vi "ForceBalanceServer.vi"() -> ()   [LabVIEW 2017]
uses:
  <vilib>/Analysis/4window.llb/windowTd.ctl
  <vilib>/measure/maspectr.llb/Power Spectrum and PSD Export Mode.ctl
  <vilib>/Analysis/baseanly.llb/Mean (DBL).vi
  <vilib>/Analysis/baseanly.llb/A x Vector.vi
  Globals/mainWTControl.vi
  <vilib>/Utility/file.llb/Write To Spreadsheet File (DBL).vi
  <vilib>/Utility/file.llb/Read From Spreadsheet File (DBL).vi
  <vilib>/measure/maspectr.llb/FFT Power Spectrum and PSD for 1 Chan.vi
  <vilib>/Analysis/NI_AALBase.lvlib
  <vilib>/measure/NI_MAPro.lvlib
  <vilib>/Analysis/NI_AALPro.lvlib
panel:
  out "PSD":cluster{"f0":dbl, "df":dbl, "magnitude":dbl[]}(graph)
  in  "Time Target (s)":dbl=100000.0
  in  "Sampling Period":dbl=0.01
  in  "Sampling Freq.":dbl=500.0
  in  "x":bool
  out "Fx                     Fy                     Fz                    Mx                   My                    Mz":dbl[](array[numeric])=[0.39367133033328505, 0.12640519158271346, -0.035168369141984894, 0.07356448847559971, 0.08928756090020755, 0.03408632169703757]
  in  "stop":bool
  out "Waveform Chart":dynamicdata(graph)=[{"t0"=timestamp(3625740071.8186145 s since 1904-01-01), "dt"=0.002, "Y"=[1.4132434446437658, 1.4869062871436736, 1.4652020568354351, 1.4342899711432204, 1.515516408827019], "attributes"=variant("NI_ChannelName"=variant(string "Voltage_0"), "NI_UnitDescription"=variant(string "Volts"))}, {"t0"=timestamp(3625740071.8186283 s since 1904-01-01), "dt"=0.002, "Y"=[0.4493782119596065, 0.441156910799936, 0.42537201251587176, 0.4112313744050537, 0.41221793055431444], "attributes"=variant("NI_ChannelName"=variant(string "Voltage_1"), "NI_UnitDescription"=variant(string "Volts"))}, {"t0"=timestamp(3625740071.818642 s since 1904-01-01), "dt"=0.002, "Y"=[0.1241435215364698, 0.13861301307479987, 0.18070607894651378, 0.13466678811720997, 0.12841859858966923], "attributes"=variant("NI_ChannelName"=variant(string "Voltage_2"), "NI_UnitDescription"=variant(string "Volts"))}, {"t0"=timestamp(3625740071.8186564 s since 1904-01-01), "dt"=0.002, "Y"=[4.929329220143692, 4.876055168157049, 4.92110791573665, 4.952020020475538, 4.8872361419192885], "attributes"=variant("NI_ChannelName"=variant(string "Voltage_3"), "NI_UnitDescription"=variant(string "Volts"))}, {"t0"=timestamp(3625740071.8186703 s since 1904-01-01), "dt"=0.002, "Y"=[1.7019754755920375, 1.6973715480570852, 1.6858617292118738, 1.741437711535304, 1.7019754755920375], "attributes"=variant("NI_ChannelName"=variant(string "Voltage_4"), "NI_UnitDescription"=variant(string "Volts"))}, {"t0"=timestamp(3625740071.8186846 s since 1904-01-01), "dt"=0.002, "Y"=[-1.6523161496933905, -1.626994516567589, -1.6023305886073516, -1.6164712405886696, -1.6292964831977657], "attributes"=variant("NI_ChannelName"=variant(string "Voltage_5"), "NI_UnitDescription"=variant(string "Volts"))}]
  out "L2                   S                  D2                  L1                  L3                  D1":dbl[](array[numeric])=[1.4630316337186229, 0.42787128804695646, 0.14130960005293253, 1.7057243879976673, 4.913149693286444, -1.6254817957309533]
  out "Amber Check":bool[](array[boolean])
  out "Amber Check Fail":bool
  out "OMFG Check":bool[](array[boolean])
  out "OMFG Check Fail":bool
  out "Mean Convergence":dbl(graph)=0.08995560655426219
  in  "Blank Button":bool
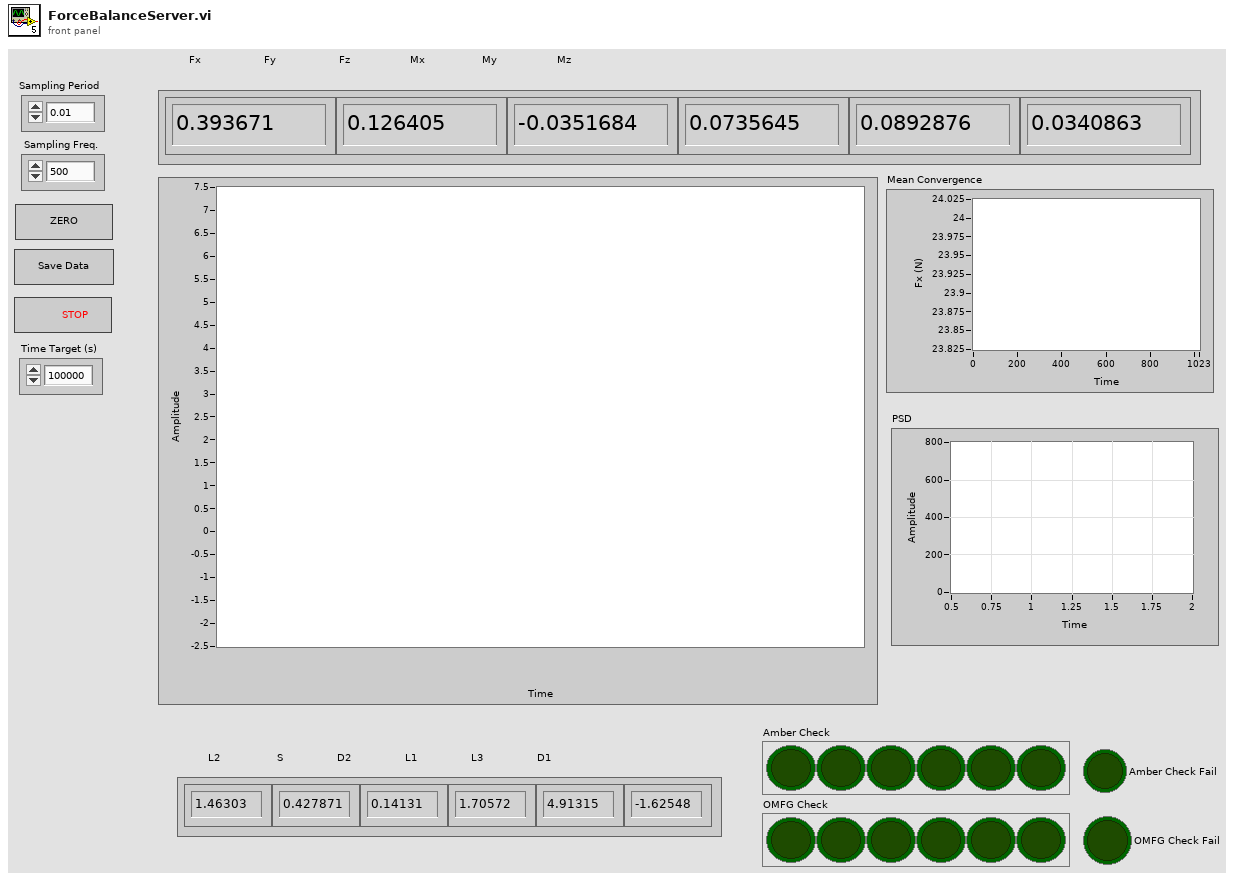
[diagram p1: front panel]
types:
  T1 = typedef "NI_MAPro.lvlib/Power Spectrum and PSD Export Mode.ctl" = u16
  T2 = typedef "NI_AALPro.lvlib/windowTd.ctl" = u32
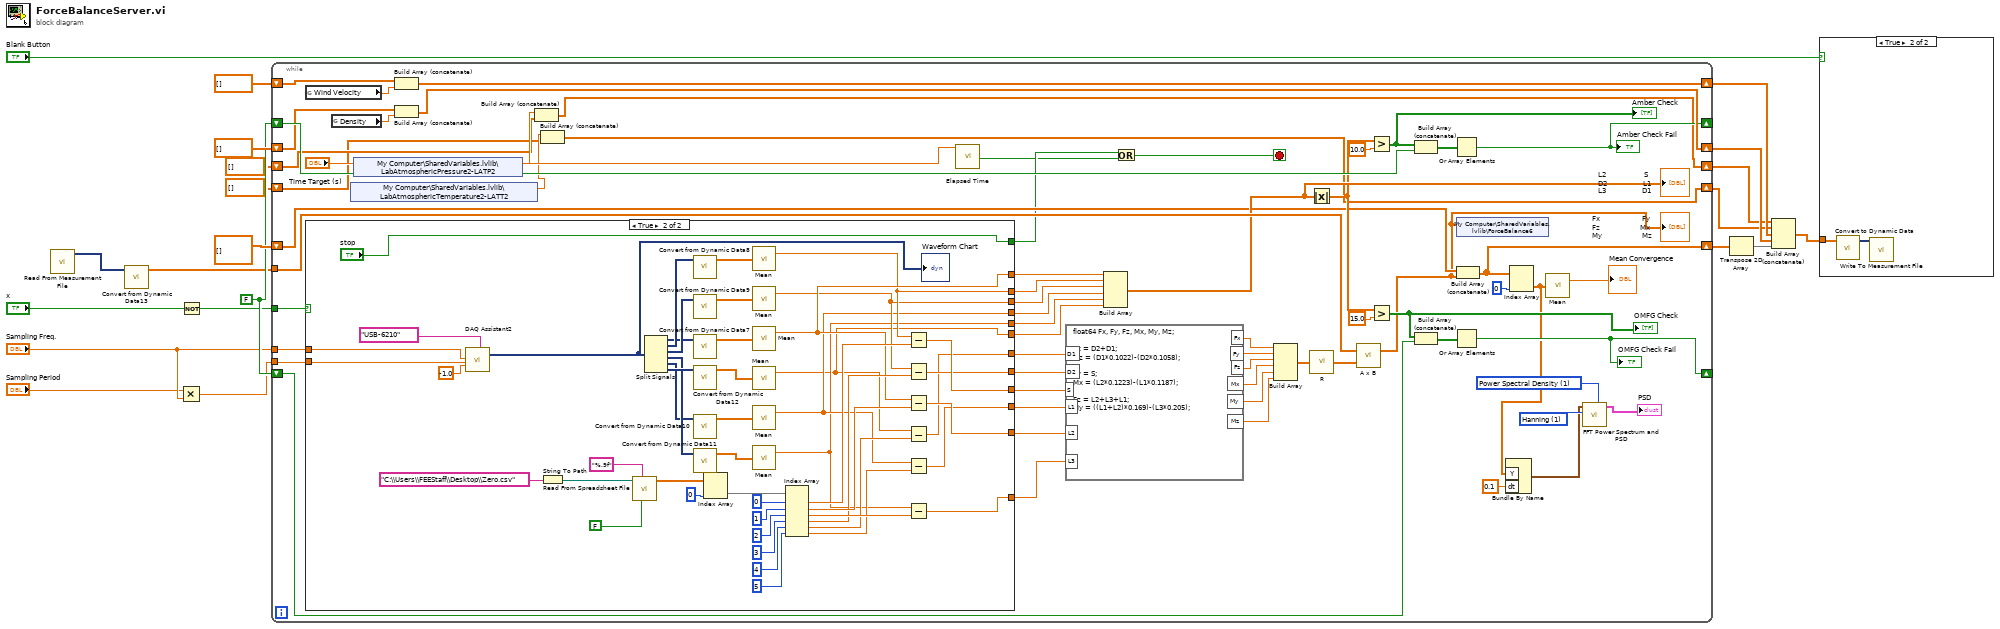
[diagram p0: block diagram]
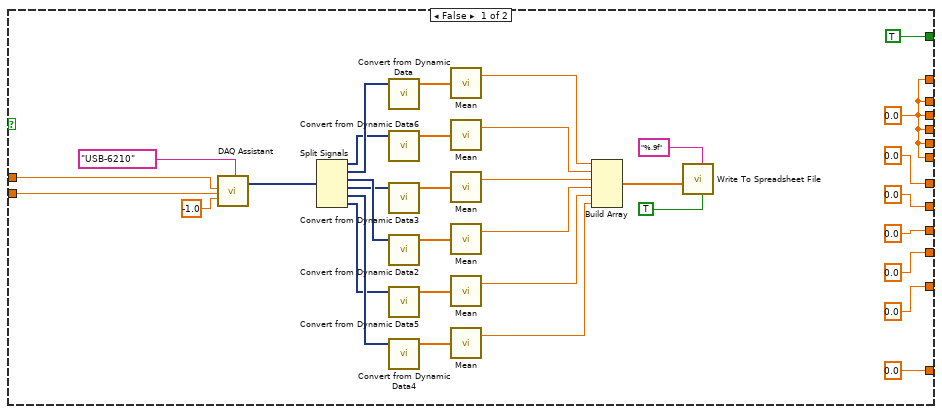
[diagram p3: hidden frame]
diagram:
  w13 = FALSE
  n1 = call "Read From Measurement File"() -> ("Signals"=w10:dynamicdata)  [unwired: 6 in, 5 out]
  n2 = call "Convert from Dynamic Data13"("Dynamic Data Type"=w10) -> ("Array"=w11:dbl[][])  [unwired: 3 in]
  n3 = Multiply(x="Sampling Period", y="Sampling Freq.") -> (x*y=w9:dbl)
  n4 = Not(x="x") -> (.not. x?=w5:bool)
  n5 = while {
    tunnel: w5 -> [w84]
    tunnel: "Sampling Freq." -> [w83]
    tunnel: w9 -> [w82]
    tunnel: w11 -> [w81]
    shift-right: [w40] -> _
    shift-left: w13 -> [w58]
    shift-right: [w41] -> _
    shift-left: w13 -> [w53]
    shift-right: [w49] -> w18
    shift-left: dbl[] [] -> [w48]
    shift-right: [w46] -> w16
    shift-left: dbl[] [] -> [w45]
    shift-right: [w42] -> w19
    shift-left: dbl[][] [] -> [w43]
    shift-right: [w31] -> w2
    shift-left: dbl[] [] -> [w32]
    shift-right: [w30] -> w1
    shift-left: dbl[] [] -> [w29]
    stop <- w36 stop-if-true
    w26 = T1 1 items=["Power Spectrum", "Power Spectral Density"] ("export mode")
    w27 = T2 1 items=["Rectangle"=0, "Hanning"=1, "Hamming"=2, "Blackman-Harris"=3, "Exact Blackman"=4, "Blackman"=5, "Flat Top"=6, "4 Term B-Harris "=7, "7 Term B-Harris"=8, "Low Sidelobe"=9, "Blackman Nuttall"=11, "Triangle"=30, "Bartlett-Hanning"=31, "Bohman"=32, "Parzen"=33, "Welch"=34, "Kaiser"=60, "Dolph-Chebyshev"=61, "Gaussian"=62] ("window")
    n6 = global read "mainWTControl.vi" "Wind Velocity"() -> (w50:dbl)
    n7 = case shown="True" w84 {
      tunnel: [0.0 w133] -> w74
      tunnel: [0.0 w132] -> w73
      tunnel: [0.0 w152] -> w77
      tunnel: [0.0 w151] -> w76
      tunnel: [0.0 w153] -> w75
      tunnel: [0.0 w154] -> w78
      tunnel: w83 -> [w118 w167]
      tunnel: w82 -> [w117 w166]
      tunnel: [TRUE ("stop") "stop"] -> w38
      tunnel: [w85 w124] -> w66
      tunnel: [w85 w123] -> w65
      tunnel: [w85 w122] -> w64
      tunnel: [w85 w121] -> w63
      tunnel: [w85 w120] -> w62
      tunnel: [w85 w119] -> w61
      frame False {
        w85 = 0.0
        n8 = call "DAQ Assistant"("rate"=w118, "number of samples"=w117, "timeout (s)"=-1.0, "device name"=tag "USB-6210") -> ("data"=w104:dynamicdata)  [unwired: 13 in, 2 out]
        n9 = Split Signals(w104) -> (w92:dynamicdata, w103:dynamicdata, w101:dynamicdata, w99:dynamicdata, w97:dynamicdata, w95:dynamicdata)  [unwired: 6 in]
        n10 = call "Convert from Dynamic Data"("Dynamic Data Type"=w103) -> ("Array"=w102:dbl[])  [unwired: 3 in]
        n11 = call "Convert from Dynamic Data6"("Dynamic Data Type"=w92) -> ("Array"=w88:dbl[])  [unwired: 3 in]
        n12 = call "Convert from Dynamic Data3"("Dynamic Data Type"=w99) -> ("Array"=w98:dbl[])  [unwired: 3 in]
        n13 = call "Convert from Dynamic Data2"("Dynamic Data Type"=w101) -> ("Array"=w100:dbl[])  [unwired: 3 in]
        n14 = call "Convert from Dynamic Data5"("Dynamic Data Type"=w95) -> ("Array"=w94:dbl[])  [unwired: 3 in]
        n15 = call "Convert from Dynamic Data4"("Dynamic Data Type"=w97) -> ("Array"=w96:dbl[])  [unwired: 3 in]
        n16 = call-poly <vilib>:"Mean.vi"("X"=w102) -> ("mean"=w109:dbl)  [unwired: 1 out]
        n17 = call-poly <vilib>:"Mean.vi"("X"=w88) -> ("mean"=w106:dbl)  [unwired: 1 out]
        n18 = call-poly <vilib>:"Mean.vi"("X"=w98) -> ("mean"=w89:dbl)  [unwired: 1 out]
        n19 = call-poly <vilib>:"Mean.vi"("X"=w100) -> ("mean"=w108:dbl)  [unwired: 1 out]
        n20 = call-poly <vilib>:"Mean.vi"("X"=w94) -> ("mean"=w107:dbl)  [unwired: 1 out]
        n21 = call-poly <vilib>:"Mean.vi"("X"=w96) -> ("mean"=w87:dbl)  [unwired: 1 out]
        n22 = Build Array(w109, w106, w89, w108, w107, w87) -> (w105:dbl[])
        n23 = call-poly <vilib>:"Write To Spreadsheet File.vi"("transpose? (no:F)"=TRUE, "format (%.3f)"="%.9f", "1D data"=w105) -> ()  [unwired: 5 in, 1 out]
      }
      frame True {
        n24 = call "DAQ Assistant2"("rate"=w167, "number of samples"=w166, "timeout (s)"=-1.0, "device name"=tag "USB-6210") -> ("data"=w125:dynamicdata)  [unwired: 12 in, 3 out]
        "Waveform Chart" <- w125
        n25 = String To Path(string="C:\\Users\\FEEStaff\\Desktop\\Zero.csv" ("format (%.3f)")) -> (path=w134:path)
        n26 = call-poly <vilib>:"Read From Spreadsheet File.vi"("transpose (no:F)"=FALSE, "format (%.3f)"="%.9f", "file path (dialog if empty)"=w134) -> ("all rows"=w157:dbl[][])  [unwired: 4 in, 4 out]
        n27 = Split Signals(w125) -> (w141:dynamicdata, w147:dynamicdata, w145:dynamicdata, w128:dynamicdata, w127:dynamicdata, w142:dynamicdata)  [unwired: 6 in]
        n28 = call "Convert from Dynamic Data8"("Dynamic Data Type"=w147) -> ("Array"=w146:dbl[])  [unwired: 3 in]
        n29 = call "Convert from Dynamic Data9"("Dynamic Data Type"=w145) -> ("Array"=w130:dbl[])  [unwired: 3 in]
        n30 = call "Convert from Dynamic Data7"("Dynamic Data Type"=w141) -> ("Array"=w148:dbl[])  [unwired: 3 in]
        n31 = call "Convert from Dynamic Data12"("Dynamic Data Type"=w142) -> ("Array"=w131:dbl[])  [unwired: 3 in]
        n32 = call "Convert from Dynamic Data10"("Dynamic Data Type"=w127) -> ("Array"=w144:dbl[])  [unwired: 3 in]
        n33 = call "Convert from Dynamic Data11"("Dynamic Data Type"=w128) -> ("Array"=w143:dbl[])  [unwired: 3 in]
        n34 = Index Array(array=w157, index (col)=0 ("disabled index (col)")) -> (element=w155:dbl[])  [unwired: 1 in]
        n35 = call-poly <vilib>:"Mean.vi"("X"=w146) -> ("mean"=w123:dbl)  [unwired: 1 out]
        n36 = call-poly <vilib>:"Mean.vi"("X"=w130) -> ("mean"=w122:dbl)  [unwired: 1 out]
        n37 = call-poly <vilib>:"Mean.vi"("X"=w148) -> ("mean"=w124:dbl)  [unwired: 1 out]
        n38 = call-poly <vilib>:"Mean.vi"("X"=w131) -> ("mean"=w119:dbl)  [unwired: 1 out]
        n39 = call-poly <vilib>:"Mean.vi"("X"=w144) -> ("mean"=w121:dbl)  [unwired: 1 out]
        n40 = call-poly <vilib>:"Mean.vi"("X"=w143) -> ("mean"=w120:dbl)  [unwired: 1 out]
        n41 = Index Array(array=w155, index #1=0 ("index (row)"), index #2=1 ("index (row)"), index #3=2 ("index (row)"), index #4=3 ("index (row)"), index #5=4 ("index (row)"), index #6=5 ("index (row)")) -> (element #1=w140:dbl, element #2=w139:dbl, element #3=w138:dbl, element #4=w137:dbl, element #5=w136:dbl, element #6=w129:dbl)
        n42 = Subtract(x=w123, y=w140) -> (x-y=w154:dbl)
        n43 = Subtract(x=w122, y=w137) -> (x-y=w133:dbl)
        n44 = Subtract(x=w124, y=w139) -> (x-y=w152:dbl)
        n45 = Subtract(x=w119, y=w136) -> (x-y=w132:dbl)
        n46 = Subtract(x=w121, y=w129) -> (x-y=w151:dbl)
        n47 = Subtract(x=w120, y=w138) -> (x-y=w153:dbl)
      }
    }
    n48 = global read "mainWTControl.vi" "Density"() -> (w47:dbl)
    n49 = shared-variable "My Computer\\SharedVariables.lvlib\\LabAtmosphericTemperature2-LATT2"() -> (w33:dbl)  [unwired: 1 in, 1 out]
    n50 = shared-variable "My Computer\\SharedVariables.lvlib\\LabAtmosphericPressure2-LATP2"() -> (w34:dbl)  [unwired: 1 in, 1 out]
    n51 = Build Array (concatenate)(w48, w50) -> (w49:dbl[])
    n52 = Build Array (concatenate)(w45, w47) -> (w46:dbl[])
    n53 = Build Array (concatenate)(w34, w32) -> (w31:dbl[])
    n54 = Build Array (concatenate)(w33, w29) -> (w30:dbl[])
    n55 = call "Elapsed Time"("Time Target (s)"="Time Target (s)") -> ("Time has Elapsed"=w37:bool)  [unwired: 11 in, 7 out]
    n56 = formula code="float64 Fx, Fy, Fz, Mx, My, Mz;\n\nFx = D2+D1;\nMz = (D1*0.1022)-(D2*0.1058);\n\nFy = S;\nMx = (L2*0.1223)-(L1*0.1187);\n\nFz = L2+L3+L1;\nMy = ((L1+L2)*0.169)-(L3*0.205);"("D1"=w73, "D2"=w74, "S"=w78, "L1"=w76, "L2"=w77, "L3"=w75) -> ("Fx"=w72:dbl, "Fy"=w71:dbl, "Fz"=w70:dbl, "Mx"=w69:dbl, "My"=w68:dbl, "Mz"=w67:dbl)
    n57 = Build Array(w66, w65, w64, w63, w62, w61) -> (w60:dbl[])
    "L2                   S                  D2                  L1                  L3                  D1" <- w60
    n58 = Or(x=w38, y=w37) -> (x .or. y?=w36:bool)
    n59 = Build Array(w72, w71, w70, w69, w68, w67) -> (w79:dbl[])
    n60 = Absolute Value(x=w60) -> (abs(x)=w55:dbl[])
    n61 = call "R.vi"("1x6"=w79) -> ("27x1"=w80:dbl[])
    n62 = call-poly <vilib>:"A x B.vi"("Vector"=w80, "A"=w81) -> ("A x Vector"=w39:dbl[])  [unwired: 1 out]
    "Fx                     Fy                     Fz                    Mx                   My                    Mz" <- w39
    n63 = Greater?(x=w55, y=10.0 ("Numeric")) -> (0:w56:bool[])
    "Amber Check" <- w56
    n64 = Greater?(x=w55, y=15.0) -> (0:w51:bool[])
    "OMFG Check" <- w51
    n65 = Build Array (concatenate)(w56, w58) -> (w57:bool[])
    n66 = Build Array (concatenate)(w51, w53) -> (w52:bool[])
    n67 = Or Array Elements(Boolean array=w57) -> (logical OR=w40:bool)
    "Amber Check Fail" <- w40
    n68 = Or Array Elements(Boolean array=w52) -> (logical OR=w41:bool)
    "OMFG Check Fail" <- w41
    n69 = shared-variable "My Computer\\SharedVariables.lvlib\\ForceBalance6"(w39) -> ()  [unwired: 1 in, 1 out]
    n70 = Build Array (concatenate)(w43, w39) -> (w42:dbl[][])
    n71 = Index Array(array=w42, index (col)=0 ("index")) -> (element=w24:dbl[])  [unwired: 1 in]
    n72 = Bundle By Name("Y"=w24, "dt"=0.1) -> (w22:waveform(dbl))  [unwired: 1 in]
    n73 = call-poly <vilib>:"Mean.vi"("X"=w24) -> ("mean"=→"Mean Convergence":dbl)  [unwired: 1 out]
    n74 = call-poly <vilib>:"FFT Power Spectrum and PSD.vi"("export mode"=w26, "window"=w27, "time signal"=w22) -> ("Power Spectrum / PSD"=→"PSD":cluster{"f0":dbl, "df":dbl, "magnitude":dbl[]})  [unwired: 5 in, 3 out]
  }
  n75 = Transpose 2D Array(2D array=w19) -> (transposed array=w20:dbl[][])
  n76 = Build Array (concatenate)(w2, w1, w18, w16, w20) -> (w21:dbl[][])
  n77 = case shown="True" "Blank Button" {
    tunnel: w21 -> [_ w169]
    frame False {
    }
    frame True {
      n78 = call "Convert to Dynamic Data"("2D Array"=w169) -> ("Dynamic Data Type"=w168:dynamicdata)  [unwired: 3 in]
      n79 = call "Write To Measurement File"("Signals"=w168) -> ()  [unwired: 16 in, 3 out]
    }
  }
